vi "Main-TempC-GCode.vi"() -> ()   [LabVIEW 2022 SP3]
uses:
  MoveSwitch.ctl
  <vilib>/Instr/_visa.llb/VISA Configure Serial Port (Instr).vi
panel:
  in  "?":T1(tab)
  in  "VISA resource":refnum<visa-resource-name>
  out "?":dbl(slide) scale=0.0..100.0
  out "humidity (%)":dbl
  out "?":dbl(slide) scale=0.0..100.0
  in  "stop":bool
  out "<Low":bool
  out "Normal":bool
  out ">High":bool
  out "Normal temperature level":dbl(slide) scale=-55.0..125.0
  in  "L 2":bool
  in  "L 3":bool
  out "Normal HumIDITY level 2":dbl(slide) scale=-55.0..125.0
  out "<Low 2":bool
  out "Normal 2":bool
  out ">High 2":bool
  in  "L 8":bool
  in  "L 9":bool
  in  "Path":path
  out "?":bool
  in  "Write to file":bool
  in  "L":bool
  out "Received data":string
  in  "H":bool
  out "Waveform Chart":cluster{dbl, dbl}(graph)
  out "Waveform Chart":cluster{dbl}(graph)
  out "Response":string
  out "History":string
  out "Command":string
  out "MoveString":string
  in  "Manual Positioning":T2
  in  "distance(mm)":dbl=5.0
  out "Local Origin":cluster{"X":dbl, "Y":dbl, "Z":dbl}
  in  "SetLocal":bool
  in  "One line Command":string
  in  "Send":bool
  in  "Machine-Home":bool
  out "M-Pos":cluster{"X":dbl, "Y":dbl, "Z":dbl}
  out "Local-Pos":cluster{"X":dbl, "Y":dbl, "Z":dbl}
  in  "Pos Button":bool
  in  "Local-Home":bool
  out "G-code list":string
  in  "Select G-code file":bool
  in  "Send G-code":bool
  in  "stop 2":bool
  out "Measure":bool
  in  "Grbl":refnum<visa-resource-name>="COM3"
  out "Connecting to":string
  out "Version":string
  # "Device control"
  # "Dalas Temperature"
  # "DHT11"
  # "HumIDITY Level properties"
  # "Temperature Level properties"
  # "Upper fan fan on"
  # "Upper fan fan off"
  # "Gas control"
  # "Gas on"
  # "Gas off"
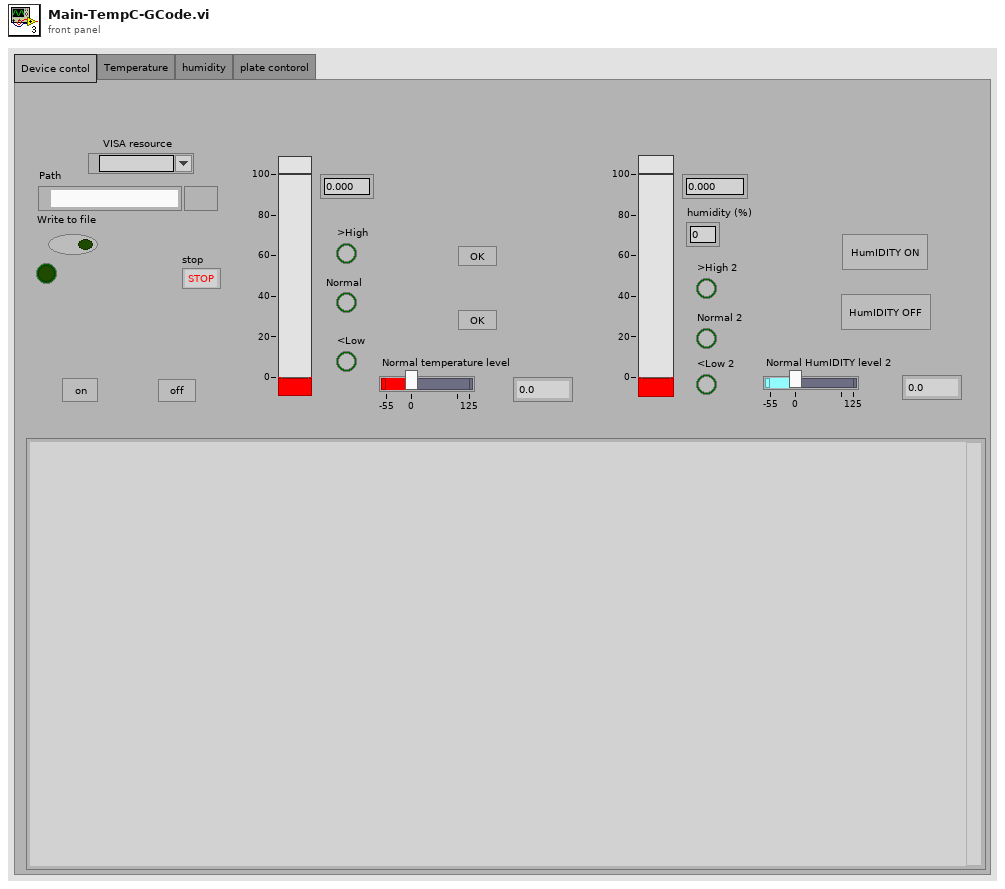
[diagram p1: front panel]
types:
  T1 = enum32{"Device contol", "Temperature", "humidity", "plate contorol"}
  T2 = typedef "MoveSwitch.ctl" = cluster{"X+":bool, "X-":bool, "Y+":bool, "Y-":bool, "Z+":bool, "Z-":bool}
  T3 = cluster{"VISA resource name":refnum<visa-resource-name>, "baud rate":u32, "data bits":u16, "parity":u16, "stop bits":u16, "flow control":u16}
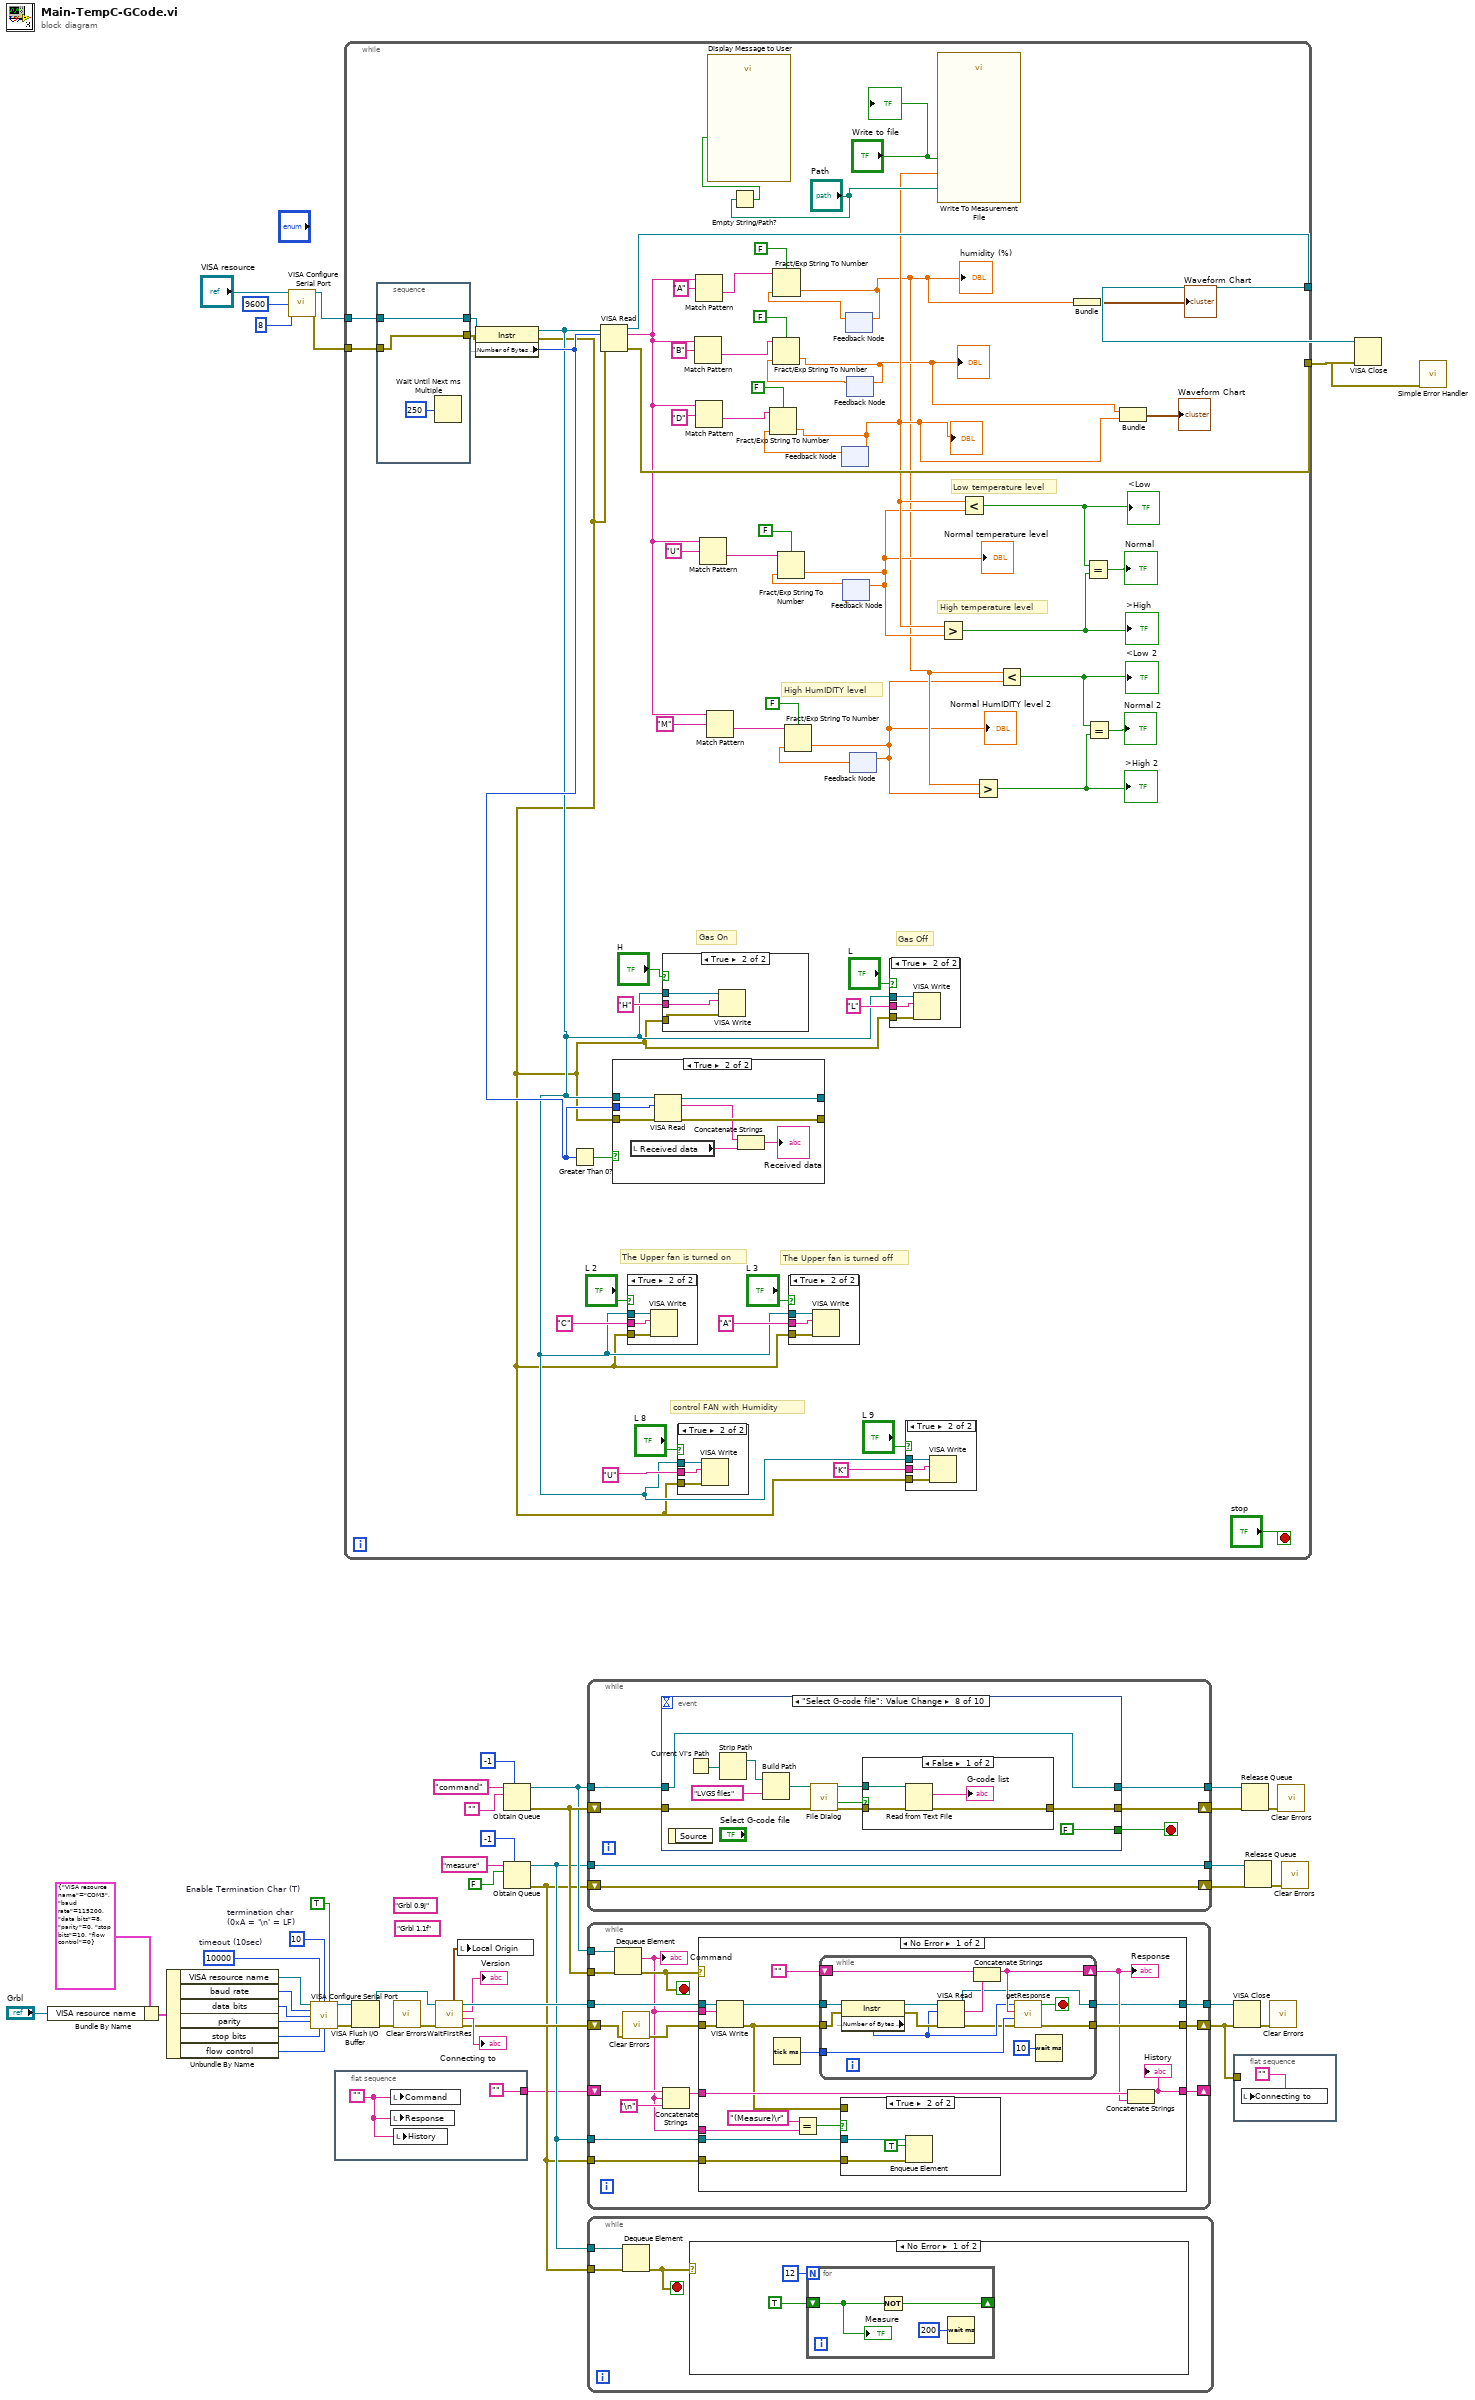
[diagram p0: block diagram]
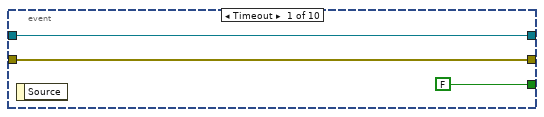
[diagram p3: hidden frame]
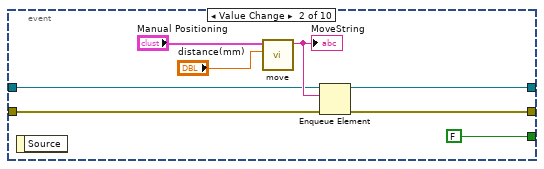
[diagram p4: hidden frame]
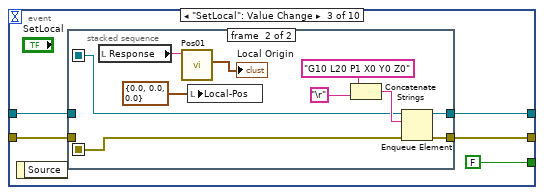
[diagram p5: hidden frame]
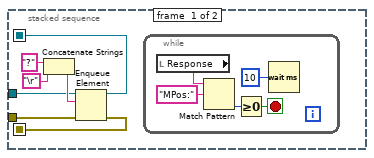
[diagram p6: hidden frame]
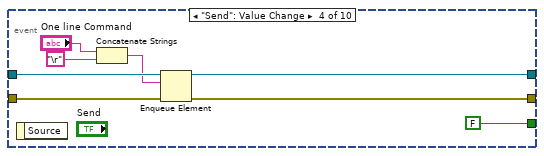
[diagram p7: hidden frame]
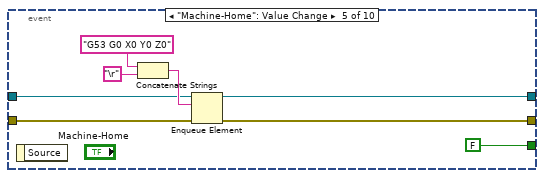
[diagram p8: hidden frame]
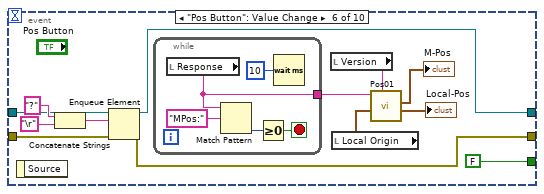
[diagram p9: hidden frame]
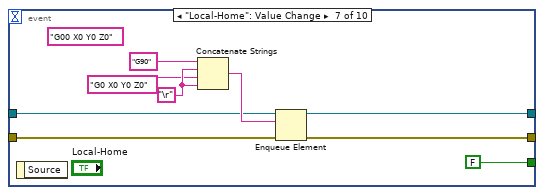
[diagram p10: hidden frame]
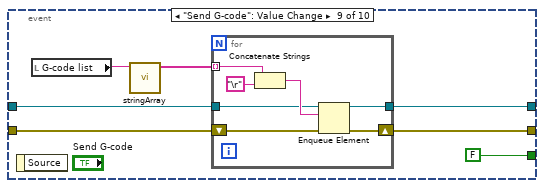
[diagram p12: hidden frame]
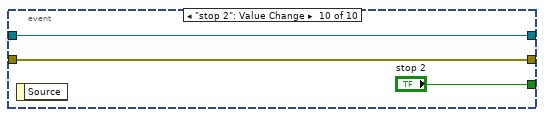
[diagram p13: hidden frame]
diagram:
  (unwired) "Grbl 1.1f" ("Version")
  (unwired) "Grbl 0.9j" ("Version")
  w20 = u8 10  # termination char (0xA = '\n' = LF)
  w31 = TRUE  # Enable Termination Char (T)
  w42 = u32 10000  # timeout (10sec)
  n1 = Bundle By Name(cluster=T3 {"VISA resource name"="COM3", "baud rate"=115200, "data bits"=8, "parity"=0, "stop bits"=10, "flow control"=0} ("COM"), "VISA resource name"="Grbl") -> (w38:T3)
  n2 = Unbundle By Name(w38) -> ("VISA resource name"=w37:refnum<visa-resource-name>, "baud rate"=w36:u32, "data bits"=w35:u16, "parity"=w34:u16, "stop bits"=w33:u16, "flow control"=w32:u16)
  n3 = call-poly "VISA Configure Serial Port"("VISA resource name"="VISA resource", "baud rate (9600)"=u32 9600, "data bits (8)"=u16 8) -> ("VISA resource name out"=w47:refnum<visa-resource-name>, "error out"=w46:errorcluster)  [unwired: 11 in]
  n4 = call-poly "VISA Configure Serial Port"("VISA resource name"=w37, "timeout (10sec)"=w42, "termination char\n(0xA = '\\n' = LF)"=w20, "Enable Termination\nChar (T)"=w31, "baud rate (9600)"=w36, "data bits (8)"=w35, "parity (0:none)"=w34, "stop bits (10: 1 bit)"=w33, "flow control (0:none)"=w32) -> ("VISA resource name out"=w29:refnum<visa-resource-name>, "error out"=w30:errorcluster)  [unwired: 1 in, 4 out]
  n5 = flat-sequence {
    tunnel: [""] -> w3
    frame #0 {
      w52 = ""
      n6 = local write "Command"(w52) -> ()
      n7 = local write "Response"(w52) -> ()
      n8 = local write "History"(w52) -> ()
    }
  }
  n9 = while {
    tunnel: w47 -> [w112]
    tunnel: w46 -> [w110]
    tunnel: [w99] -> w45
    tunnel: [w98] -> w44
    stop <- "stop" stop-if-true
    # "control FAN with Humidity"
    # "High HumIDITY level"
    # "High temperature level"
    # "Low temperature level"
    # "The Upper fan is turned off"
    # "The Upper fan is turned on"
    # "Gas Off"
    # "Gas On"
    n10 = stacked-sequence {
      tunnel: w112 -> [w143]
      tunnel: [w143] -> w111
      tunnel: w110 -> [w142]
      tunnel: [w142] -> w109
      frame #0 {
        n11 = Wait Until Next ms Multiple(millisecond multiple=u32 250) -> ()  [unwired: 1 out]
      }
    }
    n12 = property class="Instr"(reference=w111, error in=w109) -> (reference out=w63:refnum<visa-resource-name>, error out=w62:errorcluster, "Serial Settings:Number of Bytes at Serial Port"=w87:u32)
    n13 = Greater Than 0?(x=w87) -> (x > 0?=w92:bool)
    n14 = VISA Read(VISA resource name=w63, byte count=w87, error in (no error)=w62) -> (VISA resource name out=w99:refnum<visa-resource-name>, read buffer=w68:string, error out=w98:errorcluster)  [unwired: 1 out]
    n15 = case shown="True" w92 {
      tunnel: w63 -> [w132 w140]
      tunnel: w62 -> [w131 w139]
      tunnel: [w132 w138] -> _
      tunnel: [w131 w137] -> _
      tunnel: w87 -> [_ w136]
      frame False {
      }
      frame True {
        n16 = local read "Received data"() -> (w134:string)
        n17 = VISA Read(VISA resource name=w140, byte count=w136, error in (no error)=w139) -> (VISA resource name out=w138:refnum<visa-resource-name>, read buffer=w133:string, error out=w137:errorcluster)  [unwired: 1 out]
        n18 = Concatenate Strings(w133, w134) -> (→"Received data":string)
      }
    }
    n19 = case shown="True" "L 2" {
      tunnel: w63 -> [_ w124]
      tunnel: w62 -> [_ w123]
      tunnel: "C" -> [_ w122]
      frame False {
      }
      frame True {
        n20 = VISA Write(VISA resource name=w124, write buffer=w122, error in (no error)=w123) -> ()  [unwired: 3 out]
      }
    }
    n21 = case shown="True" "H" {
      tunnel: "H" -> [_ w130]
      tunnel: w63 -> [_ w129]
      tunnel: w62 -> [_ w128]
      frame False {
      }
      frame True {
        n22 = VISA Write(VISA resource name=w129, write buffer=w130, error in (no error)=w128) -> ()  [unwired: 3 out]
      }
    }
    n23 = case shown="True" "L 8" {
      tunnel: w63 -> [_ w118]
      tunnel: w62 -> [_ w117]
      tunnel: "U" -> [_ w116]
      frame False {
      }
      frame True {
        n24 = VISA Write(VISA resource name=w118, write buffer=w116, error in (no error)=w117) -> ()  [unwired: 3 out]
      }
    }
    n25 = Match Pattern(string=w68, regular expression="B") -> (after substring=w104:string)  [unwired: 1 in, 3 out]
    n26 = Match Pattern(string=w68, regular expression="A") -> (after substring=w105:string)  [unwired: 1 in, 3 out]
    n27 = Match Pattern(string=w68, regular expression="D") -> (after substring=w97:string)  [unwired: 1 in, 3 out]
    n28 = Match Pattern(string=w68, regular expression="U") -> (after substring=w76:string)  [unwired: 1 in, 3 out]
    n29 = Match Pattern(string=w68, regular expression="M") -> (after substring=w69:string)  [unwired: 1 in, 3 out]
    n30 = Empty String/Path?(string/path="Path") -> (empty?=w59:bool)
    n31 = call "Display Message to User"("Enable"=w59) -> ()  [unwired: 9 in, 2 out]
    n32 = case shown="True" "L 3" {
      tunnel: w63 -> [_ w121]
      tunnel: w62 -> [_ w120]
      tunnel: "A" -> [_ w119]
      frame False {
      }
      frame True {
        n33 = VISA Write(VISA resource name=w121, write buffer=w119, error in (no error)=w120) -> ()  [unwired: 3 out]
      }
    }
    n34 = feedback #1() -> (w95:dbl)  [unwired: 1 in]
    n35 = Fract/Exp String To Number(use system decimal point (T)=FALSE, string=w97, default (0 dbl)=w95) -> (number=w58:dbl)  [unwired: 1 in, 1 out]
    "?" <- w58
    n36 = feedback-in #1(w58) -> ()
    n37 = feedback #2() -> (w78:ext)  [unwired: 1 in]
    n38 = Fract/Exp String To Number(use system decimal point (T)=FALSE, string=w76, default (0 dbl)=w78) -> (number=w57:ext)  [unwired: 1 in, 1 out]
    "Normal temperature level" <- w57
    n39 = feedback-in #2(w57) -> ()
    n40 = feedback #3() -> (w101:dbl)  [unwired: 1 in]
    n41 = Fract/Exp String To Number(use system decimal point (T)=FALSE, string=w105, default (0 dbl)=w101) -> (number=w54:dbl)  [unwired: 1 in, 1 out]
    "humidity (%)" <- w54
    n42 = feedback-in #3(w54) -> ()
    n43 = feedback #4() -> (w100:dbl)  [unwired: 1 in]
    n44 = Fract/Exp String To Number(use system decimal point (T)=FALSE, string=w104, default (0 dbl)=w100) -> (number=w56:dbl)  [unwired: 1 in, 1 out]
    "?" <- w56
    n45 = feedback-in #4(w56) -> ()
    n46 = feedback #5() -> (w71:ext)  [unwired: 1 in]
    n47 = Fract/Exp String To Number(use system decimal point (T)=FALSE, string=w69, default (0 dbl)=w71) -> (number=w53:ext)  [unwired: 1 in, 1 out]
    "Normal HumIDITY level 2" <- w53
    n48 = feedback-in #5(w53) -> ()
    n49 = case shown="True" "L" {
      tunnel: w63 -> [_ w127]
      tunnel: w62 -> [_ w126]
      tunnel: "L" -> [_ w125]
      frame False {
      }
      frame True {
        n50 = VISA Write(VISA resource name=w127, write buffer=w125, error in (no error)=w126) -> ()  [unwired: 3 out]
      }
    }
    n51 = case shown="True" "L 9" {
      tunnel: w63 -> [_ w115]
      tunnel: w62 -> [_ w114]
      tunnel: "K" -> [_ w113]
      frame False {
      }
      frame True {
        n52 = VISA Write(VISA resource name=w115, write buffer=w113, error in (no error)=w114) -> ()  [unwired: 3 out]
      }
    }
    n53 = call "Write To Measurement File"("Signals"=w58, "Enable"="Write to file", "Filename"="Path") -> ()  [unwired: 14 in, 3 out]
    n54 = Greater?(x=w58, y=w57) -> (0:w85:bool)
    ">High" <- w85
    n55 = Less?(x=w58, y=w57) -> (x < y?=w86:bool)
    "<Low" <- w86
    n56 = Greater?(x=w54, y=w53) -> (0:w74:bool)
    ">High 2" <- w74
    n57 = Less?(x=w54, y=w53) -> (x < y?=w75:bool)
    "<Low 2" <- w75
    n58 = Bundle(w54) -> (→"Waveform Chart":cluster{dbl})  [unwired: 1 in]
    n59 = Equal?(x=w86, y=w85) -> (x = y?=→"Normal":bool)
    n60 = Equal?(x=w75, y=w74) -> (x = y?=→"Normal 2":bool)
    n61 = Bundle(w56, w58) -> (→"Waveform Chart":cluster{dbl, dbl})  [unwired: 1 in]
    "?" <- "Write to file"
  }
  n62 = VISA Flush I/O Buffer(VISA resource name=w29, error in (no error)=w30) -> (VISA resource name out=w19:refnum<visa-resource-name>, error out=w15:errorcluster)  [unwired: 1 in]
  n63 = call <vilib>:"Clear Errors.vi"("error in (no error)"=w15) -> ("error out"=w14:errorcluster)  [unwired: 5 in, 1 out]
  n64 = call "WaitFirstRes.vi"("error in (no error)"=w14, "VISA in"=w19) -> ("error out"=w13:errorcluster, "String"=→"Connecting to":string, "Version"=→"Version":string, "VISA out"=w18:refnum<visa-resource-name>, "Local Origin"=w1:cluster{"X":dbl, "Y":dbl, "Z":dbl})  [unwired: 4 in, 1 out]
  n65 = local write "Local Origin"(w1) -> ()
  n66 = Obtain Queue(max queue size (-1, unlimited)=-1, name (unnamed)="command", element data type="") -> (queue out=w16:refnum<queue>, error out=w21:errorcluster)  [unwired: 2 in, 1 out]
  n67 = Obtain Queue(max queue size (-1, unlimited)=-1, name (unnamed)="measure", element data type=FALSE) -> (queue out=w5:refnum<queue>, error out=w4:errorcluster)  [unwired: 2 in, 1 out]
  n68 = while {
    tunnel: w16 -> [w149]
    shift-right: [w147] -> w24
    shift-left: w21 -> [w148]
    tunnel: [w146] -> w23
    tunnel: [w145] -> w7
    tunnel: w5 -> [w145]
    shift-right: [w144] -> w6
    shift-left: w4 -> [w144]
    stop <- w150 stop-if-true
    n69 = event shown="[7] \"Select G-code file\": Value Change" {
      selector: _ -> [_ _ _ _ _ _ _ _ _ _]
      dyn-events: _ -> [_ _ _ _ _ _ _ _ _ _]
      timeout: _ -> [_ _ _ _ _ _ _ _ _ _]
      tunnel: [FALSE FALSE ("NewVal") FALSE ("stop") FALSE ("stop") FALSE ("stop") FALSE ("stop") FALSE ("stop") FALSE ("stop") FALSE ("stop") "stop 2"] -> w150
      tunnel: w149 -> [w151 w157 w163 w196 w197 w208 w227 w230 w251 w261]
      tunnel: w148 -> [w152 w156 w166 w195 w200 w211 w222 w231 w250 w260]
      tunnel: [w152 w155 w165 w189 w199 w206 w221 w233 w248 w260] -> w147
      tunnel: [w151 w154 w162 w190 w197 w208 w226 w230 w249 w261] -> w146
      event Timeout {
        n70 = event-data() -> ()  [unwired: 1 in, 1 out]
      }
      event Value Change {
        n71 = event-data() -> ()  [unwired: 1 in, 1 out]
        n72 = call "move.vi"("dist(mm)"="distance(mm)", "Manual Positioning"="Manual Positioning") -> ("MoveString"=w158:string)  [unwired: 9 in]
        "MoveString" <- w158
        n73 = Enqueue Element(queue=w157, element=w158, error in (no error)=w156) -> (queue out=w154:refnum<queue>, error out=w155:errorcluster)  [unwired: 1 in, 1 out]
      }
      event "SetLocal": Value Change {
        n74 = event-data() -> ()  [unwired: 1 in, 1 out]
        n75 = stacked-sequence {
          seq-local: [w168 _] -> [_ w182]
          seq-local: [w167 _] -> [_ w183]
          tunnel: w166 -> [w169 _]
          tunnel: [_ w184] -> w165
          tunnel: w163 -> [w170 _]
          tunnel: [_ w185] -> w162
          frame #0 {
            n76 = Concatenate Strings("?" ("Command 2"), "\r") -> (w171:string)
            n77 = Enqueue Element(queue=w170, element=w171, error in (no error)=w169) -> (queue out=w168:refnum<queue>, error out=w167:errorcluster)  [unwired: 1 in, 1 out]
            n78 = while {
              stop <- w176 stop-if-true
              n79 = local read "Response"() -> (w175:string)
              n80 = Match Pattern(string=w175, regular expression="MPos:") -> (offset past match=w177:i32)  [unwired: 1 in, 3 out]
              n81 = Greater Or Equal To 0?(x=w177) -> (x >= 0?=w176:bool)
              n82 = Wait (ms)(milliseconds to wait=u32 10) -> ()  [unwired: 1 out]
            }
          }
          frame #1 {
            n83 = local read "Response"() -> (w181:string)
            n84 = call "Pos01.vi"("String"=w181) -> ("M-Pos"=→"Local Origin":cluster{"X":dbl, "Y":dbl, "Z":dbl})  [unwired: 9 in, 1 out]
            n85 = local write "Local-Pos"(cluster{"X":dbl, "Y":dbl, "Z":dbl} {"X"=0.0, "Y"=0.0, "Z"=0.0} ("Local-Pos")) -> ()
            n86 = Concatenate Strings("G10 L20 P1 X0 Y0 Z0" ("format string"), "\r") -> (w187:string)
            n87 = Enqueue Element(queue=w182, element=w187, error in (no error)=w183) -> (queue out=w185:refnum<queue>, error out=w184:errorcluster)  [unwired: 1 in, 1 out]
          }
        }
      }
      event "Send": Value Change {
        n88 = event-data() -> ()  [unwired: 1 in, 1 out]
        n89 = Concatenate Strings("One line Command", "\r") -> (w191:string)
        n90 = Enqueue Element(queue=w196, element=w191, error in (no error)=w195) -> (queue out=w190:refnum<queue>, error out=w189:errorcluster)  [unwired: 1 in, 1 out]
      }
      event "Machine-Home": Value Change {
        n91 = event-data() -> ()  [unwired: 1 in, 1 out]
        n92 = Concatenate Strings("G53 G0 X0 Y0 Z0" ("Command 2"), "\r") -> (w201:string)
        n93 = Enqueue Element(queue=w197, element=w201, error in (no error)=w200) -> (error out=w199:errorcluster)  [unwired: 1 in, 2 out]
      }
      event "Pos Button": Value Change {
        n94 = event-data() -> ()  [unwired: 1 in, 1 out]
        n95 = Concatenate Strings("?" ("Command 2"), "\r") -> (w212:string)
        n96 = Enqueue Element(queue=w208, element=w212, error in (no error)=w211) -> (error out=w206:errorcluster)  [unwired: 1 in, 2 out]
        n97 = while {
          tunnel: [w216] -> w207
          stop <- w217 stop-if-true
          n98 = local read "Response"() -> (w216:string)
          n99 = Match Pattern(string=w216, regular expression="MPos:") -> (offset past match=w218:i32)  [unwired: 1 in, 3 out]
          n100 = Greater Or Equal To 0?(x=w218) -> (x >= 0?=w217:bool)
          n101 = Wait (ms)(milliseconds to wait=u32 10) -> ()  [unwired: 1 out]
        }
        n102 = local read "Version"() -> (w204:string)
        n103 = local read "Local Origin"() -> (w205:cluster{"X":dbl, "Y":dbl, "Z":dbl})
        n104 = call "Pos01.vi"("Version"=w204, "Local Origin"=w205, "String"=w207) -> ("W-Pos"=→"Local-Pos":cluster{"X":dbl, "Y":dbl, "Z":dbl}, "M-Pos"=→"M-Pos":cluster{"X":dbl, "Y":dbl, "Z":dbl})  [unwired: 7 in]
      }
      event "Local-Home": Value Change {
        (unwired) "G00 X0 Y0 Z0" ("Command 2")
        w225 = "\r"
        n105 = event-data() -> ()  [unwired: 1 in, 1 out]
        n106 = Concatenate Strings("G90" ("Command 2"), w225, "G0 X0 Y0 Z0" ("Command 2"), w225) -> (w228:string)
        n107 = Enqueue Element(queue=w227, element=w228, error in (no error)=w222) -> (queue out=w226:refnum<queue>, error out=w221:errorcluster)  [unwired: 1 in, 1 out]
      }
      event "Select G-code file": Value Change {
        n108 = event-data() -> ()  [unwired: 1 in, 1 out]
        n109 = Current VI's Path() -> (path=w240:path)
        n110 = Strip Path(path=w240) -> (stripped path=w239:path)  [unwired: 1 out]
        n111 = Build Path(base path=w239, name or relative path="LVGS files") -> (appended path=w237:path)
        n112 = call "File Dialog"("start path"=w237, "error in"=w231) -> ("selected path"=w235:path, "cancelled"=w236:bool, "error out"=w234:errorcluster)  [unwired: 10 in, 1 out]
        n113 = case shown="False" w236 {
          tunnel: w235 -> [w244 _]
          tunnel: w234 -> [w242 w245]
          tunnel: [w241 w245] -> w233
          frame False {
            n114 = Read from Text File(file (use dialog)=w244, error in=w242) -> (text=→"G-code list":string, error out=w241:errorcluster)  [unwired: 2 in, 2 out]
          }
          frame True {
          }
        }
      }
      event "Send G-code": Value Change {
        n115 = event-data() -> ()  [unwired: 1 in, 1 out]
        n116 = local read "G-code list"() -> (w252:string)
        n117 = call "stringArray.vi"("CNC strings"=w252) -> ("stringArray"=w247:string[])  [unwired: 10 in]
        n118 = for {
          tunnel: w251 -> [w257]
          tunnel: [w255] -> w249
          shift-right: [w254] -> w248
          shift-left: w250 -> [w256]
          tunnel: w247 -> [w253] mode=indexing
          n119 = Concatenate Strings(w253, "\r") -> (w258:string)
          n120 = Enqueue Element(queue=w257, element=w258, error in (no error)=w256) -> (queue out=w255:refnum<queue>, error out=w254:errorcluster)  [unwired: 1 in, 1 out]
        }
      }
      event "stop 2": Value Change {
        n121 = event-data() -> ()  [unwired: 1 in, 1 out]
      }
    }
  }
  n122 = while {
    tunnel: w18 -> [w276]
    shift-right: [w271] -> w12
    shift-left: w13 -> [w268]
    tunnel: [w272] -> w41
    shift-right: [w273] -> _
    shift-left: w3 -> [w275]
    tunnel: w16 -> [w277]
    tunnel: w21 -> [w270]
    tunnel: w5 -> [w264]
    tunnel: w4 -> [w263]
    stop <- w269 stop-if-true
    n123 = Dequeue Element(queue=w277, error in (no error)=w270) -> (element=w265:string, error out=w269:errorcluster)  [unwired: 1 in, 2 out]
    "Command" <- w265
    n124 = call <vilib>:"Clear Errors.vi"("error in (no error)"=w268) -> ("error out"=w267:errorcluster)  [unwired: 5 in, 1 out]
    n125 = Concatenate Strings(w275, w265, "\n") -> (w274:string)
    n126 = case shown="No Error" w269 {
      tunnel: w276 -> [w294 w313]
      tunnel: w265 -> [w292 _]
      tunnel: w274 -> [w289 w312]
      tunnel: [w288 w312] -> w273
      tunnel: [w278 w313] -> w272
      tunnel: [w291 w314] -> w271
      tunnel: w267 -> [w290 w314]
      tunnel: w265 -> [w279 _]
      tunnel: w264 -> [w282 _]
      tunnel: w263 -> [w281 _]
      frame No Error {
        n127 = VISA Write(VISA resource name=w294, write buffer=w292, error in (no error)=w290) -> (VISA resource name out=w293:refnum<visa-resource-name>, error out=w280:errorcluster)  [unwired: 1 out]
        n128 = Tick Count (ms)() -> (millisecond timer value=w285:u32)
        n129 = Equal?(x="(Measure)\r" ("y"), y=w279) -> (x = y?=w283:bool)
        n130 = while {
          tunnel: w293 -> [w311]
          tunnel: w280 -> [w299]
          shift-right: [w306] -> w286
          shift-left: "" -> [w308]
          tunnel: [w298] -> w278
          tunnel: [w301] -> w291
          tunnel: w285 -> [w305]
          stop <- w303 stop-if-true
          n131 = property class="Instr"(reference=w311, error in=w299) -> (reference out=w309:refnum<visa-resource-name>, error out=w310:errorcluster, "Serial Settings:Number of Bytes at Serial Port"=w304:u32)
          n132 = VISA Read(VISA resource name=w309, byte count=w304, error in (no error)=w310) -> (VISA resource name out=w298:refnum<visa-resource-name>, read buffer=w307:string, error out=w302:errorcluster)  [unwired: 1 out]
          n133 = Concatenate Strings(w308, w307) -> (w306:string)
          n134 = call "getResponse.vi"("error in (no error)"=w302, "ST"=w305, "string"=w306, "Bytes at Serial Port"=w304) -> ("error out"=w301:errorcluster, "done"=w303:bool)  [unwired: 5 in, 1 out]
          n135 = Wait (ms)(milliseconds to wait=u32 10) -> ()  [unwired: 1 out]
        }
        "Response" <- w286
        n136 = case shown="True" w283 {
          tunnel: w282 -> [_ w297]
          tunnel: w281 -> [_ w296]
          tunnel: w280 -> [_ _]
          frame False {
          }
          frame True {
            n137 = Enqueue Element(queue=w297, element=TRUE, error in (no error)=w296) -> ()  [unwired: 1 in, 3 out]
          }
        }
        n138 = Concatenate Strings(w289, w286) -> (w288:string)
        "History" <- w288
      }
      frame Error {
      }
    }
  }
  n139 = while {
    tunnel: w5 -> [w317]
    tunnel: w4 -> [w316]
    stop <- w315 stop-if-true
    n140 = Dequeue Element(queue=w317, error in (no error)=w316) -> (error out=w315:errorcluster)  [unwired: 1 in, 3 out]
    n141 = case shown="No Error" w315 {
      frame No Error {
        n142 = for {
          N: 12 -> [_]
          shift-right: [w321] -> _
          shift-left: TRUE ("OPERATION") -> [w322]
          n143 = Not(x=w322) -> (.not. x?=w321:bool)
          n144 = Wait (ms)(milliseconds to wait=u32 200) -> ()  [unwired: 1 out]
          "Measure" <- w322
        }
      }
      frame Error {
      }
    }
  }
  n145 = VISA Close(VISA resource name=w41, error in (no error)=w12) -> (error out=w28:errorcluster)
  n146 = flat-sequence {
    tunnel: w12 -> [_]
    frame #0 {
      n147 = local write "Connecting to"("") -> ()
    }
  }
  n148 = Release Queue(queue=w23, error in (no error)=w24) -> (error out=w22:errorcluster)  [unwired: 1 in, 2 out]
  n149 = Release Queue(queue=w7, error in (no error)=w6) -> (error out=w8:errorcluster)  [unwired: 1 in, 2 out]
  n150 = call <vilib>:"Clear Errors.vi"("error in (no error)"=w28) -> ()  [unwired: 5 in, 2 out]
  n151 = call <vilib>:"Clear Errors.vi"("error in (no error)"=w22) -> ()  [unwired: 5 in, 2 out]
  n152 = call <vilib>:"Clear Errors.vi"("error in (no error)"=w8) -> ()  [unwired: 5 in, 2 out]
  n153 = VISA Close(VISA resource name=w45, error in (no error)=w44) -> (error out=w43:errorcluster)
  n154 = call <vilib>:"Simple Error Handler.vi"("error in (no error)"=w43) -> ()  [unwired: 4 in, 5 out]
